vi "decay detector.vi"() -> ()   [LabVIEW 2015]
uses:
  <vilib>/platform/TimedLoop/XDataNode/XDataNode.xnode
  <vilib>/Platform/TimedLoop/XDataNode/nitl_modes.ctl
  <vilib>/Platform/TimedLoop/XDataNode/XDNodeRunTimeDep.lvlib
  <vilib>/Platform/TimedLoop/XDataNode/wakeup.ctl
  <vilib>/Platform/TimedLoop/XDataNode/timing_clust.ctl
  <vilib>/Utility/file.llb/Write Delimited Spreadsheet (I64).vi
  <vilib>/Analysis/NI_AALBase.lvlib
panel:
  out "histogram":i32[](graph)
  in  "histogram bins":i32=100
  out "count rate vs time":i32[](graph)
  out "# of bins":i32
  in  "Run time (s)":i32=240
  out "counts per second":dbl(knob) scale=0.0..10.0
  in  "Bin time (ms)":i32=1000
  in  "stop":bool=TRUE
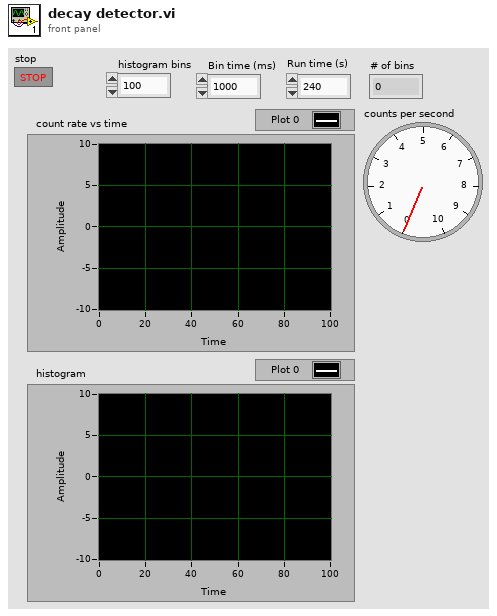
[diagram p1: front panel]
types:
  T1 = typedef "XDNodeRunTimeDep.lvlib/timing_clust.ctl" = cluster{"Expected End [f-1]":u64, "Actual End [f-1]":u64, "Finished Late? [f-1]":bool, "Expected End [i-1]":u64, "Actual End [i-1]":u64, "Finished Late? [i-1]":bool, "Expected Start [i]":u64, "Actual Start [i]":u64, "Expected Start [f]":u64, "Actual Start [f]":u64, "Source Name":string, "Structure Name":string, "Period":i64, "Deadline":i64, "Offset":i64, "Start":i64, "Priority":i32, "Timeout":i32, "Mode":T2, "Wakeup Reason":T3, "Error":errorcluster, "Source Type":string, "Secondary Source Type":string, "Global End Time":u64, "Global Start Time":u64, "Frame Duration":u64, "Iteration Duration":u64, "Assigned CPU":i32, "I/O Scan Engine Mode":u32}
  T2 = typedef "XDNodeRunTimeDep.lvlib/nitl_modes.ctl" = enum32{"No Change", "Process missed periods, maintain original phase", "Discard missed periods, maintain original phase", "Process missed periods, ignore original phase", "Discard missed periods, ignore original phase"}
  T3 = typedef "XDNodeRunTimeDep.lvlib/wakeup.ctl" = enum32{"Normal", "Aborted", "Asynchronous wakeup", "Timing source error", "Timed loop error", "Timeout"}
  T4 = cluster{"X Values":dbl[], "Histogram: h(x)":i32[]}
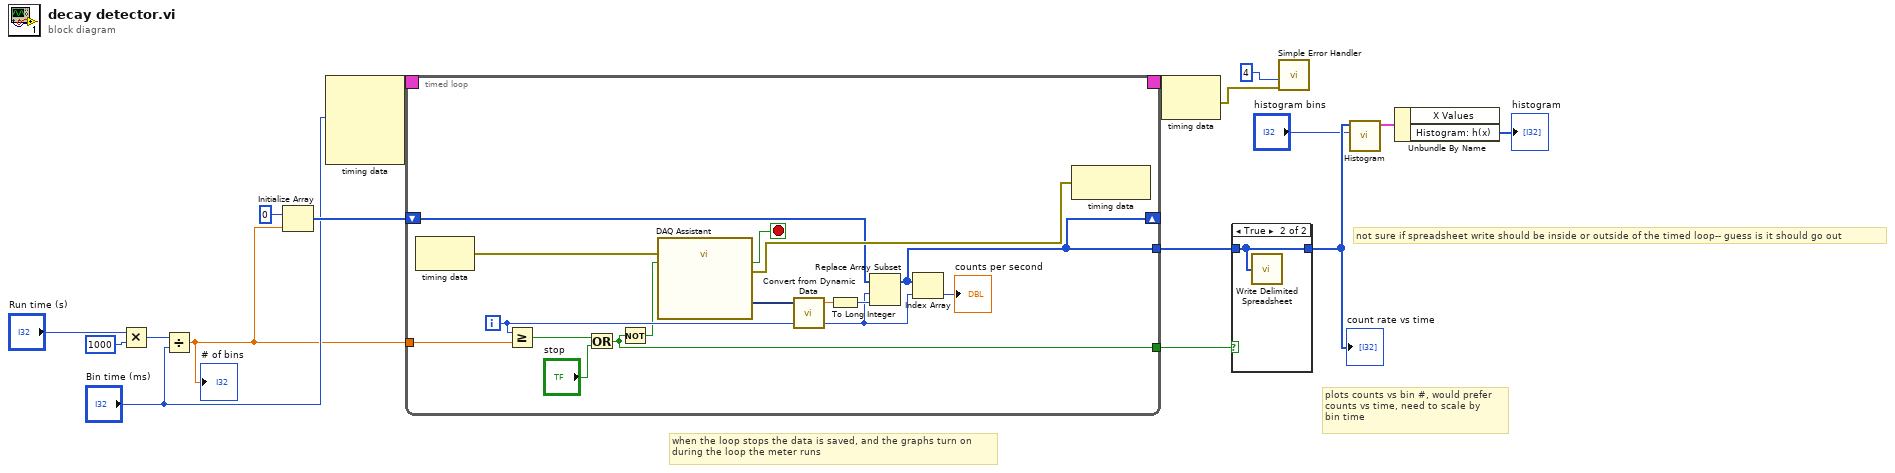
[diagram p0: block diagram]
diagram:
  # "when the loop stops the data is saved, and the graphs turn on\nduring the loop the meter runs"
  # "plots counts vs bin #, would prefer\ncounts vs time, need to scale by \nbin time"
  # "not sure if spreadsheet write should be inside or outside of the timed loop-- guess is it should go out"
  n1 = Multiply(x="Run time (s)", y=1000) -> (x*y=w10:i32)
  n2 = Divide(x=w10, y="Bin time (ms)") -> (x/y=w9:dbl)
  "# of bins" <- w9
  n3 = Initialize Array(0, w9) -> (w14:i32[])
  n4 = node-c288("Bin time (ms)") -> (w17:T1)  [unwired: 3 in]
  n5 = timed-loop {
    timing: w17 -> [_]
    timing-out: [_] -> w16
    shift-right: [w18] -> _
    shift-left: w14 -> [w27]
    tunnel: w9 -> [w24]
    tunnel: [w19] -> w8
    tunnel: [w18] -> w7
    i -> [w25]
    stop <- w21 stop-if-true
    n6 = node-c288() -> (w32:errorcluster)  [unwired: 1 in]
    n7 = Greater Or Equal?(x=w25, y=w24) -> (x >= y?=w23:bool)
    n8 = Or(x=w23, y="stop") -> (x .or. y?=w19:bool)
    n9 = Not(x=w19) -> (.not. x?=w20:bool)
    n10 = call "DAQ Assistant"("error in"=w32, "stop (F)"=w20) -> ("data"=w30:dynamicdata, "stopped"=w21:bool, "error out"=w31:errorcluster)  [unwired: 14 in, 1 out]
    n11 = call "Convert from Dynamic Data"("Dynamic Data Type"=w30) -> ("Scalar"=w29:dbl)  [unwired: 3 in]
    n12 = To Long Integer(number=w29) -> (32bit integer=w28:i32)
    n13 = Replace Array Subset(array=w27, new element=w28, index=w25) -> (w18:i32[])
    n14 = Index Array(array=w18, index=w25) -> (element=→"counts per second":i32)
    n15 = node-c288(w31) -> ()  [unwired: 1 out]
  }
  n16 = node-c288(w16) -> (w2:errorcluster)
  n17 = case shown="True" w8 {
    tunnel: w7 -> [_ w38]
    tunnel: [_ w38] -> w6
    frame False {
    }
    frame True {
      n18 = call-poly <vilib>:"Write Delimited Spreadsheet.vi"("1D data"=w38) -> ()  [unwired: 13 in, 2 out]
    }
  }
  "count rate vs time" <- w6
  n19 = call <vilib>:"Simple Error Handler.vi"("type of dialog (OK msg:1)"=4, "error in (no error)"=w2) -> ()  [unwired: 3 in, 5 out]
  n20 = call <vilib>:"Histogram.vi"("intervals"="histogram bins", "X"=w6) -> ("Histogram Graph"=w4:T4)  [unwired: 6 in, 3 out]
  n21 = Unbundle By Name(w4) -> ("Histogram: h(x)"=→"histogram":i32[])  [unwired: 1 out]
